vi "Read Roles.vi"(8 "error in (no error)":errorcluster, 11 "GoalKickAllyPlayVSS in":refnum<class "GoalKickAllyPlayVSS.lvclass">) -> (0 "error out":errorcluster, 2 "Roles":T1, 3 "GoalKickAllyPlayVSS out":refnum<class "GoalKickAllyPlayVSS.lvclass">)   [LabVIEW 2020, in "GoalKickAllyPlayVSS.lvclass"]
uses:
  GoalKickAllyPlayVSS.lvclass
  HaltRole_class/HaltRole.lvclass
  GoAndKickRoleVSS_class/GoAndKickRoleVSS.lvclass
  GoalKickAllyPlayVSS.lvclass/GoalKickAllyPlayVSS.ctl
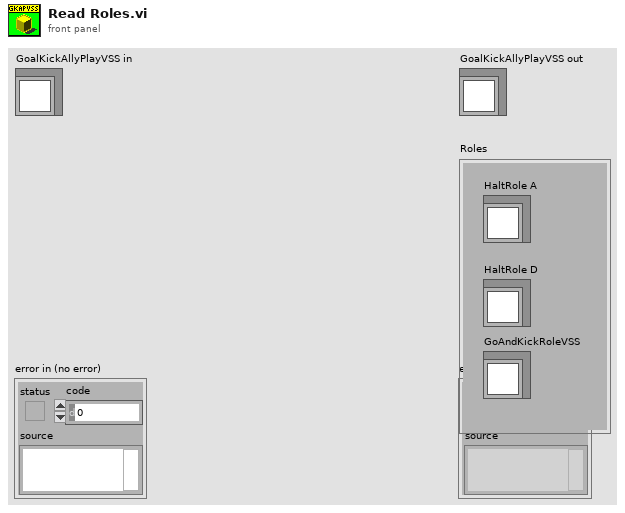
[diagram p1: front panel]
types:
  T1 = cluster{"HaltRole A":refnum<class "HaltRole.lvclass">, "GoAndKickRoleVSS":refnum<class "GoAndKickRoleVSS.lvclass">, "HaltRole D":refnum<class "HaltRole.lvclass">}
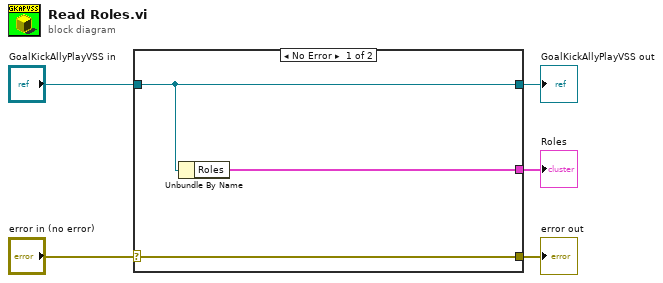
[diagram p0: block diagram]
diagram:
  n1 = case shown="No Error" "error in (no error)" {
    selector: "error in (no error)" -> [w8 w9]
    tunnel: [w8 w9] -> w4
    tunnel: [w7 w10] -> w2
    tunnel: "GoalKickAllyPlayVSS in" -> [w7 w10]
    tunnel: [w6 _] -> w1
    frame No Error {
      n2 = Unbundle By Name(w7) -> ("Roles"=w6:T1)
    }
    frame Error {
    }
  }
  "error out" <- w4
  "GoalKickAllyPlayVSS out" <- w2
  "Roles" <- w1
